vi "Sign Message.vi"(7 "Message In":T1, 11 "Error In":errorcluster) -> (4 "Signature":string, 8 "Message Out":T1, 15 "Error Out":errorcluster)   [LabVIEW 2023, in "Message Handler.lvclass"]
uses:
  Message Handler.lvclass
  Interfaces/ICanCommunicate/Message.ctl
  <vilib>/security/Message Digest/API/Instances/Byte Array/SHA-256 Byte Array Checksum.vi
  Message Handler.lvclass/Message Handler.ctl
  <vilib>/security/Message Digest/API/NI_Message Digest API.lvlib
  Interfaces/ICanCommunicate/ICanCommunicate.lvclass
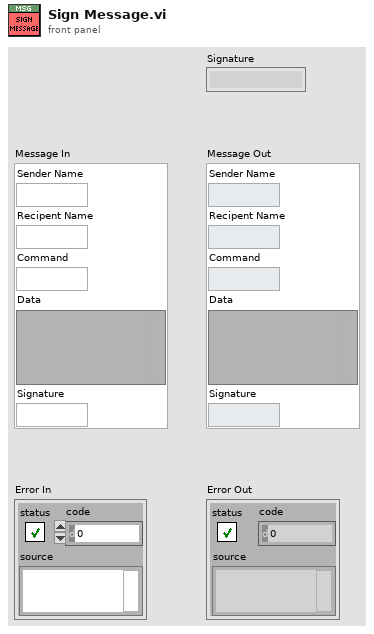
[diagram p1: front panel]
types:
  T1 = typedef "ICanCommunicate.lvclass/Message.ctl" = cluster{"Sender Name":string, "Recipent Name":string, "Command":string, "Data":variant, "Signature":string}
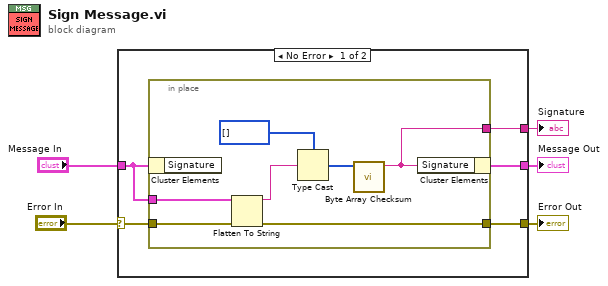
[diagram p0: block diagram]
diagram:
  n1 = case shown="No Error" "Error In" {
    selector: "Error In" -> [w10 w18]
    tunnel: [w9 w18] -> w4
    tunnel: "Message In" -> [w8 _]
    tunnel: [w7 _] -> w2
    tunnel: [w6 _] -> w1
    frame No Error {
      n2 = in-place {
        in-place-border: w10 -> [w14]
        in-place-border: [w13] -> w9
        in-place-border: w8 -> [w12]
        in-place-border: [w11] -> w6
        n3 = in-place-cluster #1(w8) -> ()  [unwired: 1 out]
        n4 = Flatten To String(anything=w12, error in (no error)=w14) -> (data string=w16:string, error out=w13:errorcluster)  [unwired: 2 in, 1 out]
        n5 = Type Cast(type=u8[] [], x=w16) -> (*(type *) &x=w15:u8[])
        n6 = call-poly <vilib>:"Byte Array Checksum.vi"("buffer"=w15) -> ("digest"=w11:string)  [unwired: 10 in]
        n7 = in-place-cluster #1("Signature"=w11) -> (w7:T1)
      }
    }
    frame Error {
    }
  }
  "Error Out" <- w4
  "Message Out" <- w2
  "Signature" <- w1
